vi "BuildFarm Installer.vi"   [LabVIEW 2017]
panel:
  # "BuildFarm installation..."
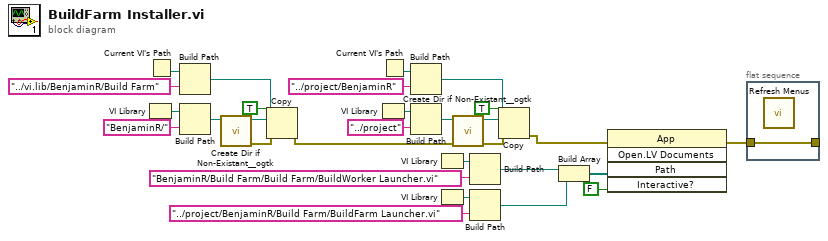
[diagram p0: block diagram]
diagram:
  n1 = VI Library() -> (path=w25:path)
  n2 = Current VI's Path() -> (path=w29:path)
  n3 = Build Path(base path=w29, name or relative path="../vi.lib/BenjaminR/Build Farm") -> (appended path=w23:path)
  n4 = Build Path(base path=w25, name or relative path="BenjaminR/") -> (appended path=w22:path)
  n5 = call <userlib>:"Create Dir if Non-Existant__ogtk.vi"("Directory Path"=w22) -> ("error out"=w21:errorcluster, "dup Directory Path"=w11:path)  [unwired: 8 in, 1 out]
  n6 = Copy(8:w21, 9:TRUE ("overwrite (F)"), 10:w11, 11:w23) -> (0:w15:errorcluster)  [unwired: 1 in, 2 out]
  n7 = VI Library() -> (path=w20:path)
  n8 = Current VI's Path() -> (path=w26:path)
  n9 = Build Path(base path=w26, name or relative path="../project/BenjaminR") -> (appended path=w16:path)
  n10 = Build Path(base path=w20, name or relative path="../project") -> (appended path=w17:path)
  n11 = VI Library() -> (path=w3:path)
  n12 = VI Library() -> (path=w5:path)
  n13 = call <userlib>:"Create Dir if Non-Existant__ogtk.vi"("error in (no error)"=w15, "Directory Path"=w17) -> ("error out"=w12:errorcluster, "dup Directory Path"=w18:path)  [unwired: 7 in, 1 out]
  n14 = Build Path(base path=w3, name or relative path="BenjaminR/Build Farm/Build Farm/BuildWorker Launcher.vi") -> (appended path=w1:path)
  n15 = Build Path(base path=w5, name or relative path="../project/BenjaminR/Build Farm/BuildFarm Launcher.vi") -> (appended path=w4:path)
  n16 = Copy(8:w12, 9:TRUE ("overwrite (F)"), 10:w18, 11:w16) -> (0:w9:errorcluster)  [unwired: 1 in, 2 out]
  n17 = Build Array(w1, w4) -> (w8:path[])
  n18 = invoke class="App" method="Open.LV Documents"(error in=w9, "Path"=w8, "Interactive?"=FALSE) -> (error out=w10:errorcluster)  [unwired: 2 in, 4 out]
  n19 = flat-sequence {
    tunnel: w10 -> [w30]
    tunnel: [w30] -> _
    frame #0 {
      n20 = call <resource>:"Refresh Menus.vi"() -> ()  [unwired: 12 in]
    }
  }
